vi "PH.vi"(8 "error in (no error)":errorcluster, 10 "Axis Number":i32, 11 "Agilis in":T2) -> (0 "error out":errorcluster, 1 "Limit Status":T1 items=["Both inactive", "Ch1 active", "Ch2 active", "Both active"], 2 "Triggered?":bool, 3 "Agilis out":T2)   [LabVIEW 2016, in "Drivers.lvlib" / "Agilis.lvlib"]
doc: "This command is specific to AG-UC8. The piezo actuators are selected by paris which are grouped in four channels. This command <b>query</b> the selected channel."
uses:
  Agilis.lvlib
  AgilisCmdLib Refnum.ctl
  D:/Trace Grabber/Drivers/Agilis/AgilisCmdLib.dll
  AgilisCmdLib.dll
  Limit Status.ctl
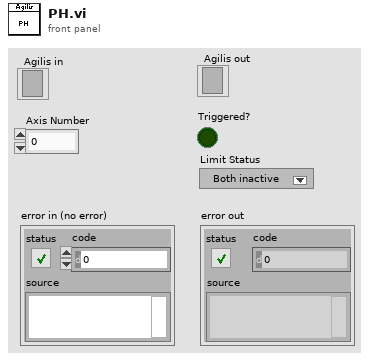
[diagram p1: front panel]
types:
  T1 = typedef "Drivers.lvlib/Agilis.lvlib/Limit Status.ctl" = i32
  T2 = typedef "Drivers.lvlib/Agilis.lvlib/AgilisCmdLib Refnum.ctl" = refnum<k24>
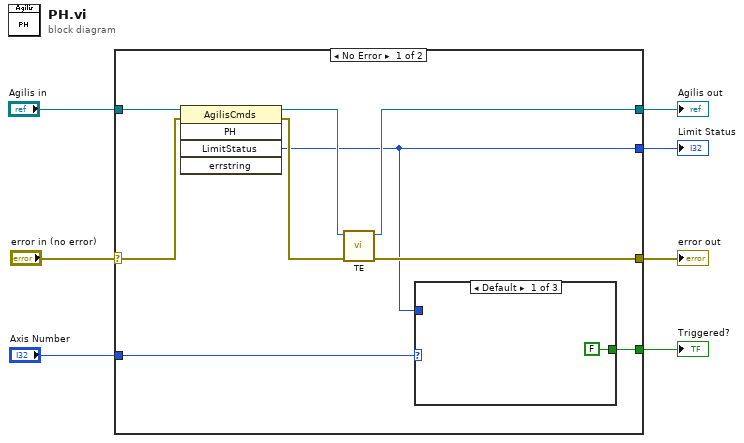
[diagram p0: block diagram]
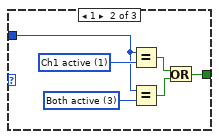
[diagram p2: hidden frame]
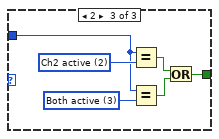
[diagram p3: hidden frame]
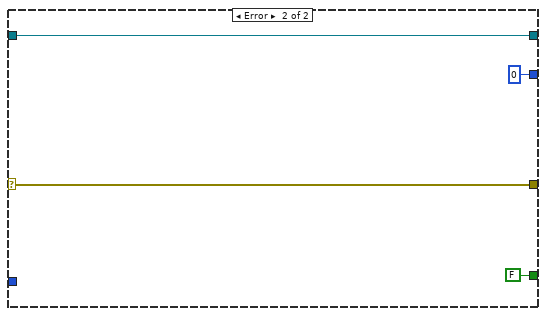
[diagram p4: hidden frame]
diagram:
  n1 = case shown="No Error" "error in (no error)" {
    selector: "error in (no error)" -> [w15 w33]
    tunnel: "Agilis in" -> [w16 w32]
    tunnel: [w11 w32] -> w5
    tunnel: [w13 w33] -> w4
    tunnel: [w10 0 ("LimitStatus")] -> w3
    tunnel: "Axis Number" -> [w9 _]
    tunnel: [w8 FALSE] -> w1
    frame No Error {
      n2 = invoke class="AgilisCmds" method="PH"(reference=w16, error in=w15) -> (reference out=w12:T2, error out=w14:errorcluster, "LimitStatus"=w10:i32)  [unwired: 3 in, 2 out]
      n3 = call "TE.vi"("error in (no error)"=w14, "Agilis in"=w12) -> ("error out"=w13:errorcluster, "Agilis out"=w11:T2)  [unwired: 8 in]
      n4 = case shown="Default" w9 {
        tunnel: w10 -> [_ w22 w28]
        tunnel: [FALSE w18 w24] -> w8
        frame Default {
        }
        frame 1 {
          w21 = T1 3 items=["Both inactive", "Ch1 active", "Ch2 active", "Both active"] ("y")
          w23 = T1 1 items=["Both inactive", "Ch1 active", "Ch2 active", "Both active"] ("y")
          n5 = Equal?(x=w22, y=w23) -> (x = y?=w20:bool)
          n6 = Equal?(x=w22, y=w21) -> (x = y?=w19:bool)
          n7 = Or(x=w20, y=w19) -> (x .or. y?=w18:bool)
        }
        frame 2 {
          w27 = T1 3 items=["Both inactive", "Ch1 active", "Ch2 active", "Both active"] ("y")
          w29 = T1 2 items=["Both inactive", "Ch1 active", "Ch2 active", "Both active"] ("y")
          n8 = Equal?(x=w28, y=w29) -> (x = y?=w26:bool)
          n9 = Equal?(x=w28, y=w27) -> (x = y?=w25:bool)
          n10 = Or(x=w26, y=w25) -> (x .or. y?=w24:bool)
        }
      }
    }
    frame Error {
    }
  }
  "Agilis out" <- w5
  "error out" <- w4
  "Limit Status" <- w3
  "Triggered?" <- w1
